vi "cameraFrame.vi"() -> (0 "x轴旋转引用":refnum<vi>, 1 "y轴旋转引用":refnum<vi>, 2 "z轴旋转引用":refnum<vi>, 3 "相机引用":refnum<vi>)   [LabVIEW 2012]
uses:
  <vilib>/picture/3D Picture Control/NI_3D Picture Control.lvlib
panel:
  in  "z轴旋转":sgl caption="角"
  in  "y轴旋转":sgl caption="角"
  in  "x轴旋转":sgl caption="角"
  in  "停止 2":bool
  out "三维图片 2":refnum<vi>(3d-picture)
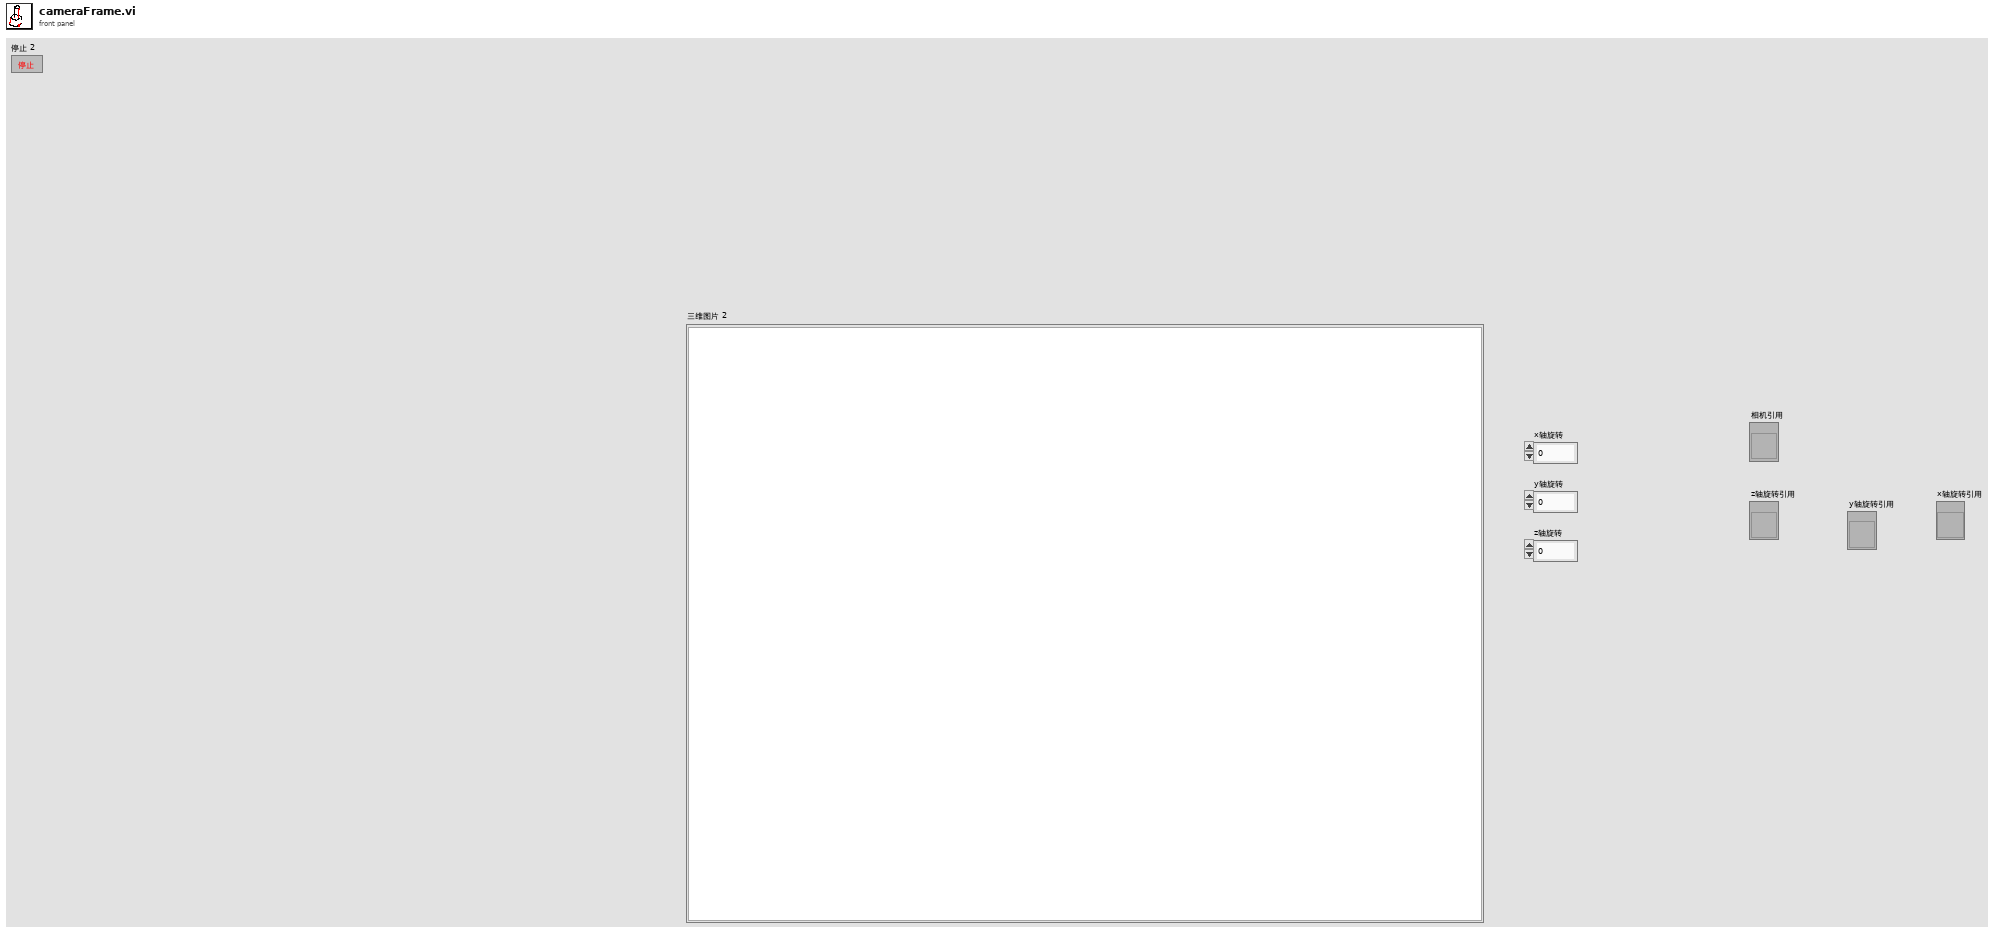
[diagram p1: front panel]
types:
  T1 = cluster{"Red":sgl, "Green":sgl, "Blue":sgl, "Alpha":sgl}
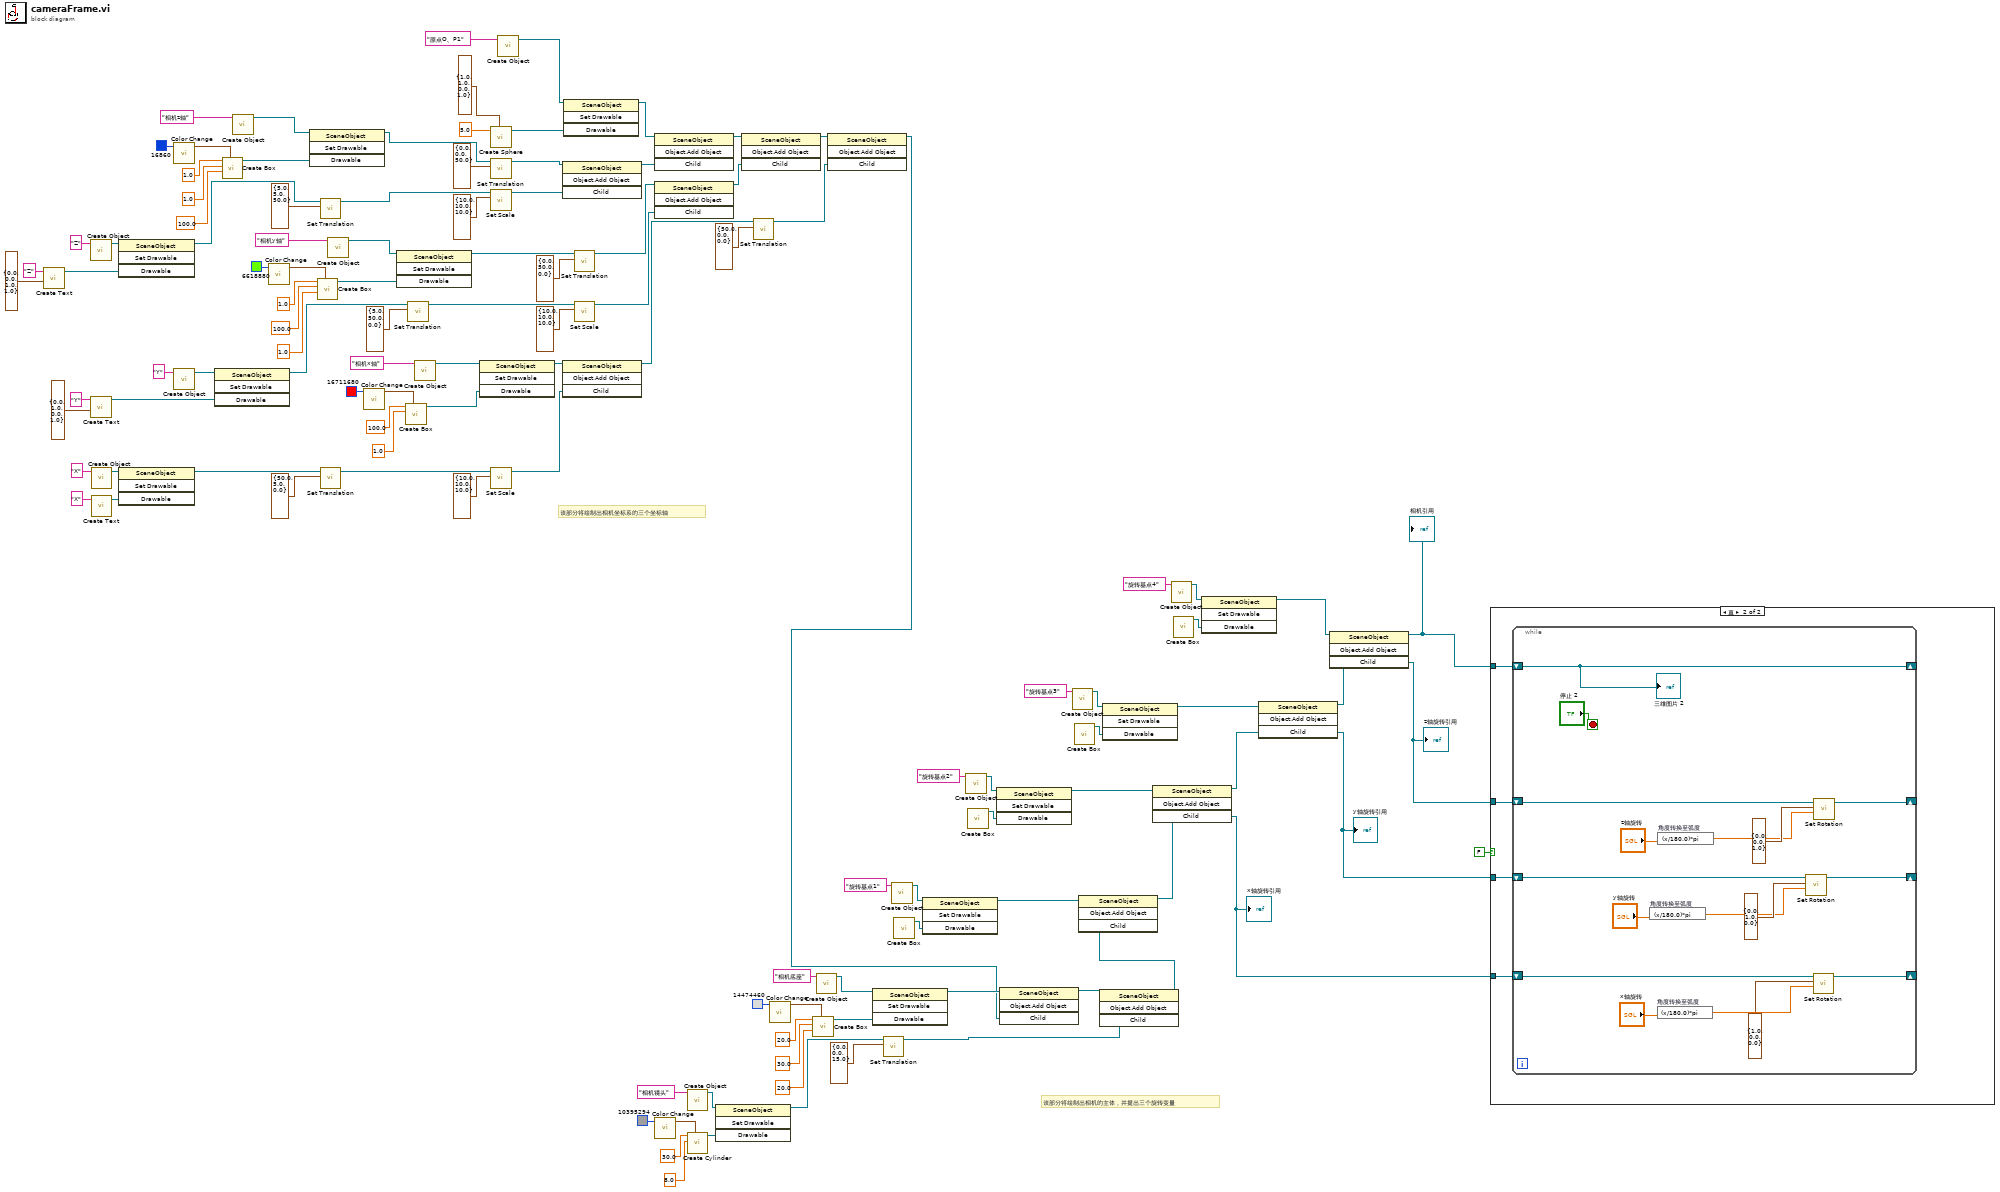
[diagram p0: block diagram]
diagram:
  # "该部分将绘制出相机的主体，并提出三个旋转变量"
  # "该部分将绘制出相机坐标系的三个坐标轴"
  n1 = call <vilib>:"Create Text.vi"("Color"=T1 {"Red"=0.0, "Green"=0.0, "Blue"=1.0, "Alpha"=1.0}, "Text"="Z") -> ("New Text Refnum"=w38:refnum<vi>)  [unwired: 8 in, 1 out]
  n2 = call <vilib>:"Create Object.vi"("Name"="Z") -> ("Scene:New Object"=w39:refnum<vi>)  [unwired: 9 in, 1 out]
  n3 = call <vilib>:"Create Text.vi"("Color"=T1 {"Red"=0.0, "Green"=1.0, "Blue"=0.0, "Alpha"=1.0}, "Text"="Y") -> ("New Text Refnum"=w50:refnum<vi>)  [unwired: 8 in, 1 out]
  n4 = call <vilib>:"Create Object.vi"("Name"="X") -> ("Scene:New Object"=w64:refnum<vi>)  [unwired: 9 in, 1 out]
  n5 = call <vilib>:"Create Text.vi"("Text"="X") -> ("New Text Refnum"=w63:refnum<vi>)  [unwired: 9 in, 1 out]
  n6 = invoke class="SceneObject" method="Set Drawable"(reference=w39, "Drawable"=w38) -> (reference out=w37:refnum<vi>)  [unwired: 2 in, 3 out]
  n7 = invoke class="SceneObject" method="Set Drawable"(reference=w64, "Drawable"=w63) -> (reference out=w59:refnum<vi>)  [unwired: 2 in, 3 out]
  n8 = call <vilib>:"Color Change.vi"("Color"=u32 16860) -> ("RGBA"=w98:cluster{"R":sgl, "G":sgl, "B":sgl, "A":sgl})  [unwired: 10 in]
  n9 = call <vilib>:"Create Object.vi"("Name"="Y") -> ("Scene:New Object"=w51:refnum<vi>)  [unwired: 9 in, 1 out]
  n10 = invoke class="SceneObject" method="Set Drawable"(reference=w51, "Drawable"=w50) -> (reference out=w49:refnum<vi>)  [unwired: 2 in, 3 out]
  n11 = call <vilib>:"Create Box.vi"("Color"=w98, "Length Z"=sgl 100.0, "Length Y"=sgl 1.0, "Length X"=sgl 1.0) -> ("New Box Refnum"=w94:refnum<vi>)  [unwired: 6 in, 1 out]
  n12 = call <vilib>:"Create Object.vi"("Name"="相机z轴") -> ("Scene:New Object"=w95:refnum<vi>)  [unwired: 9 in, 1 out]
  n13 = call <vilib>:"Color Change.vi"("Color"=u32 6618880) -> ("RGBA"=w108:cluster{"R":sgl, "G":sgl, "B":sgl, "A":sgl})  [unwired: 10 in]
  n14 = invoke class="SceneObject" method="Set Drawable"(reference=w95, "Drawable"=w94) -> (reference out=w92:refnum<vi>)  [unwired: 2 in, 3 out]
  n15 = call <vilib>:"Create Box.vi"("Color"=w108, "Length Z"=sgl 1.0, "Length Y"=sgl 100.0, "Length X"=sgl 1.0) -> ("New Box Refnum"=w104:refnum<vi>)  [unwired: 6 in, 1 out]
  n16 = call <vilib>:"Set Translation.vi"("Translation"=cluster{"X":sgl, "Y":sgl, "Z":sgl} {"X"=5.0, "Y"=5.0, "Z"=50.0}, "Scene Object"=w37) -> ("Translated Object"=w35:refnum<vi>)  [unwired: 8 in, 1 out]
  n17 = call <vilib>:"Set Translation.vi"("Translation"=cluster{"X":sgl, "Y":sgl, "Z":sgl} {"X"=50.0, "Y"=5.0, "Z"=0.0}, "Scene Object"=w59) -> ("Translated Object"=w57:refnum<vi>)  [unwired: 8 in, 1 out]
  n18 = call <vilib>:"Create Object.vi"("Name"="相机y轴") -> ("Scene:New Object"=w105:refnum<vi>)  [unwired: 9 in, 1 out]
  n19 = call <vilib>:"Color Change.vi"("Color"=u32 16711680) -> ("RGBA"=w54:cluster{"R":sgl, "G":sgl, "B":sgl, "A":sgl})  [unwired: 10 in]
  n20 = invoke class="SceneObject" method="Set Drawable"(reference=w105, "Drawable"=w104) -> (reference out=w102:refnum<vi>)  [unwired: 2 in, 3 out]
  n21 = call <vilib>:"Create Box.vi"("Color"=w54, "Length Y"=sgl 1.0, "Length X"=sgl 100.0) -> ("New Box Refnum"=w113:refnum<vi>)  [unwired: 7 in, 1 out]
  n22 = call <vilib>:"Set Translation.vi"("Translation"=cluster{"X":sgl, "Y":sgl, "Z":sgl} {"X"=5.0, "Y"=50.0, "Z"=0.0}, "Scene Object"=w49) -> ("Translated Object"=w47:refnum<vi>)  [unwired: 8 in, 1 out]
  n23 = call <vilib>:"Create Object.vi"("Name"="相机x轴") -> ("Scene:New Object"=w114:refnum<vi>)  [unwired: 9 in, 1 out]
  n24 = invoke class="SceneObject" method="Set Drawable"(reference=w114, "Drawable"=w113) -> (reference out=w62:refnum<vi>)  [unwired: 2 in, 3 out]
  n25 = call <vilib>:"Create Sphere.vi"("Color"=T1 {"Red"=1.0, "Green"=1.0, "Blue"=0.0, "Alpha"=1.0}, "Radius"=sgl 5.0 ("Length X")) -> ("New Sphere Refnum"=w91:refnum<vi>)  [unwired: 8 in, 1 out]
  n26 = call <vilib>:"Set Translation.vi"("Translation"=cluster{"X":sgl, "Y":sgl, "Z":sgl} {"X"=0.0, "Y"=0.0, "Z"=50.0}, "Scene Object"=w92) -> ("Translated Object"=w31:refnum<vi>)  [unwired: 8 in, 1 out]
  n27 = call <vilib>:"Set Scale.vi"("Scale"=cluster{"X":sgl, "Y":sgl, "Z":sgl} {"X"=10.0, "Y"=10.0, "Z"=10.0}, "Scene Object"=w35) -> ("Scaled Object"=w32:refnum<vi>)  [unwired: 8 in, 1 out]
  n28 = call <vilib>:"Set Scale.vi"("Scale"=cluster{"X":sgl, "Y":sgl, "Z":sgl} {"X"=10.0, "Y"=10.0, "Z"=10.0}, "Scene Object"=w57) -> ("Scaled Object"=w56:refnum<vi>)  [unwired: 8 in, 1 out]
  n29 = call <vilib>:"Create Object.vi"("Name"="原点O、P1") -> ("Scene:New Object"=w90:refnum<vi>)  [unwired: 9 in, 1 out]
  n30 = invoke class="SceneObject" method="Object.Add Object"(reference=w31, "Child"=w32) -> (reference out=w30:refnum<vi>)  [unwired: 2 in, 3 out]
  n31 = invoke class="SceneObject" method="Object.Add Object"(reference=w62, "Child"=w56) -> (reference out=w61:refnum<vi>)  [unwired: 2 in, 3 out]
  n32 = invoke class="SceneObject" method="Set Drawable"(reference=w90, "Drawable"=w91) -> (reference out=w86:refnum<vi>)  [unwired: 2 in, 3 out]
  n33 = call <vilib>:"Set Translation.vi"("Translation"=cluster{"X":sgl, "Y":sgl, "Z":sgl} {"X"=0.0, "Y"=50.0, "Z"=0.0}, "Scene Object"=w102) -> ("Translated Object"=w44:refnum<vi>)  [unwired: 8 in, 1 out]
  n34 = call <vilib>:"Set Scale.vi"("Scale"=cluster{"X":sgl, "Y":sgl, "Z":sgl} {"X"=10.0, "Y"=10.0, "Z"=10.0}, "Scene Object"=w47) -> ("Scaled Object"=w42:refnum<vi>)  [unwired: 8 in, 1 out]
  n35 = invoke class="SceneObject" method="Object.Add Object"(reference=w86, "Child"=w30) -> (reference out=w85:refnum<vi>)  [unwired: 2 in, 3 out]
  n36 = invoke class="SceneObject" method="Object.Add Object"(reference=w44, "Child"=w42) -> (reference out=w43:refnum<vi>)  [unwired: 2 in, 3 out]
  n37 = call <vilib>:"Color Change.vi"("Color"=u32 10395294) -> ("RGBA"=w75:cluster{"R":sgl, "G":sgl, "B":sgl, "A":sgl})  [unwired: 10 in]
  n38 = call <vilib>:"Create Object.vi"("Name"="相机镜头") -> ("Scene:New Object"=w78:refnum<vi>)  [unwired: 9 in, 1 out]
  n39 = call <vilib>:"Create Cylinder.vi"("Color"=w75, "Radius"=sgl 8.0, "Height"=sgl 30.0) -> ("New Cylinder Refnum"=w79:refnum<vi>)  [unwired: 7 in, 1 out]
  n40 = invoke class="SceneObject" method="Set Drawable"(reference=w78, "Drawable"=w79) -> (reference out=w71:refnum<vi>)  [unwired: 2 in, 3 out]
  n41 = invoke class="SceneObject" method="Object.Add Object"(reference=w85, "Child"=w43) -> (reference out=w84:refnum<vi>)  [unwired: 2 in, 3 out]
  n42 = call <vilib>:"Set Translation.vi"("Translation"=cluster{"X":sgl, "Y":sgl, "Z":sgl} {"X"=50.0, "Y"=0.0, "Z"=0.0}, "Scene Object"=w61) -> ("Translated Object"=w60:refnum<vi>)  [unwired: 8 in, 1 out]
  n43 = call <vilib>:"Color Change.vi"("Color"=u32 14474460) -> ("RGBA"=w80:cluster{"R":sgl, "G":sgl, "B":sgl, "A":sgl})  [unwired: 10 in]
  n44 = call <vilib>:"Create Box.vi"("Color"=w80, "Length Z"=sgl 20.0, "Length Y"=sgl 30.0, "Length X"=sgl 20.0) -> ("New Box Refnum"=w83:refnum<vi>)  [unwired: 6 in, 1 out]
  n45 = call <vilib>:"Create Object.vi"("Name"="相机底座") -> ("Scene:New Object"=w68:refnum<vi>)  [unwired: 9 in, 1 out]
  n46 = invoke class="SceneObject" method="Object.Add Object"(reference=w84, "Child"=w60) -> (reference out=w1:refnum<vi>)  [unwired: 2 in, 3 out]
  n47 = invoke class="SceneObject" method="Set Drawable"(reference=w68, "Drawable"=w83) -> (reference out=w3:refnum<vi>)  [unwired: 2 in, 3 out]
  n48 = call <vilib>:"Set Translation.vi"("Translation"=cluster{"X":sgl, "Y":sgl, "Z":sgl} {"X"=0.0, "Y"=0.0, "Z"=15.0}, "Scene Object"=w71) -> ("Translated Object"=w14:refnum<vi>)  [unwired: 8 in, 1 out]
  n49 = call <vilib>:"Create Object.vi"("Name"="旋转基点1") -> ("Scene:New Object"=w27:refnum<vi>)  [unwired: 9 in, 1 out]
  n50 = call <vilib>:"Create Box.vi"() -> ("New Box Refnum"=w28:refnum<vi>)  [unwired: 10 in, 1 out]
  n51 = invoke class="SceneObject" method="Set Drawable"(reference=w27, "Drawable"=w28) -> (reference out=w26:refnum<vi>)  [unwired: 2 in, 3 out]
  n52 = call <vilib>:"Create Object.vi"("Name"="旋转基点2") -> ("Scene:New Object"=w23:refnum<vi>)  [unwired: 9 in, 1 out]
  n53 = call <vilib>:"Create Box.vi"() -> ("New Box Refnum"=w24:refnum<vi>)  [unwired: 10 in, 1 out]
  n54 = invoke class="SceneObject" method="Set Drawable"(reference=w23, "Drawable"=w24) -> (reference out=w22:refnum<vi>)  [unwired: 2 in, 3 out]
  n55 = invoke class="SceneObject" method="Object.Add Object"(reference=w3, "Child"=w1) -> (reference out=w2:refnum<vi>)  [unwired: 2 in, 3 out]
  n56 = call <vilib>:"Create Object.vi"("Name"="旋转基点3") -> ("Scene:New Object"=w19:refnum<vi>)  [unwired: 9 in, 1 out]
  n57 = call <vilib>:"Create Box.vi"() -> ("New Box Refnum"=w20:refnum<vi>)  [unwired: 10 in, 1 out]
  n58 = invoke class="SceneObject" method="Object.Add Object"(reference=w2, "Child"=w14) -> (reference out=w13:refnum<vi>)  [unwired: 2 in, 3 out]
  n59 = invoke class="SceneObject" method="Object.Add Object"(reference=w26, "Child"=w13) -> (reference out=w17:refnum<vi>)  [unwired: 2 in, 3 out]
  n60 = invoke class="SceneObject" method="Set Drawable"(reference=w19, "Drawable"=w20) -> (reference out=w18:refnum<vi>)  [unwired: 2 in, 3 out]
  n61 = invoke class="SceneObject" method="Object.Add Object"(reference=w22, "Child"=w17) -> (reference out=w16:refnum<vi>, "Child"=w9:refnum<vi>)  [unwired: 2 in, 2 out]
  "x轴旋转引用" <- w9
  n62 = call <vilib>:"Create Object.vi"("Name"="旋转基点4") -> ("Scene:New Object"=w5:refnum<vi>)  [unwired: 9 in, 1 out]
  n63 = call <vilib>:"Create Box.vi"() -> ("New Box Refnum"=w6:refnum<vi>)  [unwired: 10 in, 1 out]
  n64 = invoke class="SceneObject" method="Set Drawable"(reference=w5, "Drawable"=w6) -> (reference out=w4:refnum<vi>)  [unwired: 2 in, 3 out]
  n65 = invoke class="SceneObject" method="Object.Add Object"(reference=w18, "Child"=w16) -> (reference out=w15:refnum<vi>, "Child"=w10:refnum<vi>)  [unwired: 2 in, 2 out]
  "y轴旋转引用" <- w10
  n66 = invoke class="SceneObject" method="Object.Add Object"(reference=w4, "Child"=w15) -> (reference out=w12:refnum<vi>, "Child"=w11:refnum<vi>)  [unwired: 2 in, 2 out]
  "相机引用" <- w12
  "z轴旋转引用" <- w11
  n67 = case shown="真" FALSE {
    tunnel: w12 -> [_ w122]
    tunnel: w11 -> [_ w121]
    tunnel: w10 -> [_ w120]
    tunnel: w9 -> [_ w119]
    frame False {
    }
    frame True {
      n68 = while {
        shift-right: [w129] -> _
        shift-left: w121 -> [w130]
        shift-right: [w127] -> _
        shift-left: w120 -> [w128]
        shift-right: [w125] -> _
        shift-left: w119 -> [w126]
        shift-right: [w124] -> _
        shift-left: w122 -> [w124]
        stop <- "停止 2" stop-if-true
        n69 = expression code="(x/180.0)*pi" "角度转换至弧度"("y轴旋转") -> (w134:sgl)
        n70 = expression code="(x/180.0)*pi" "角度转换至弧度"("x轴旋转") -> (w137:sgl)
        n71 = expression code="(x/180.0)*pi" "角度转换至弧度"("z轴旋转") -> (w131:sgl)
        n72 = call <vilib>:"Set Rotation.vi"("Angle"=w134, "Axis"=cluster{"X":sgl, "Y":sgl, "Z":sgl} {"X"=0.0, "Y"=1.0, "Z"=0.0}, "Scene Object"=w128) -> ("Rotated Scene Object"=w127:refnum<vi>)  [unwired: 7 in, 1 out]
        n73 = call <vilib>:"Set Rotation.vi"("Angle"=w137, "Axis"=cluster{"X":sgl, "Y":sgl, "Z":sgl} {"X"=1.0, "Y"=0.0, "Z"=0.0}, "Scene Object"=w126) -> ("Rotated Scene Object"=w125:refnum<vi>)  [unwired: 7 in, 1 out]
        n74 = call <vilib>:"Set Rotation.vi"("Angle"=w131, "Axis"=cluster{"X":sgl, "Y":sgl, "Z":sgl} {"X"=0.0, "Y"=0.0, "Z"=1.0}, "Scene Object"=w130) -> ("Rotated Scene Object"=w129:refnum<vi>)  [unwired: 7 in, 1 out]
        "三维图片 2" <- w124
      }
    }
  }
